vi "TestStand - SetLVFeatureTogglesForBuildAndExecute.vi"(8 "error in":errorcluster, 11 "enable":bool) -> (0 "error out":errorcluster)   [LabVIEW 2023]
panel:
  out "previous value of UseModdateToCheckSourceChanges.Enabled":bool
  out "previous value of AppBuilder.ExportAlwaysIncludedItemsFromPPL":bool
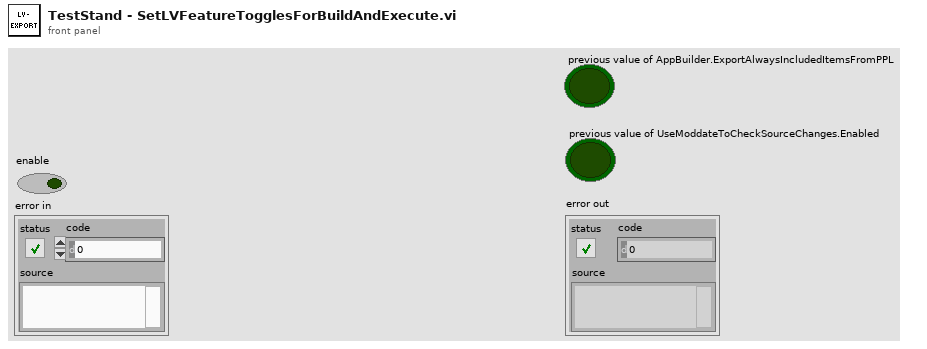
[diagram p1: front panel]
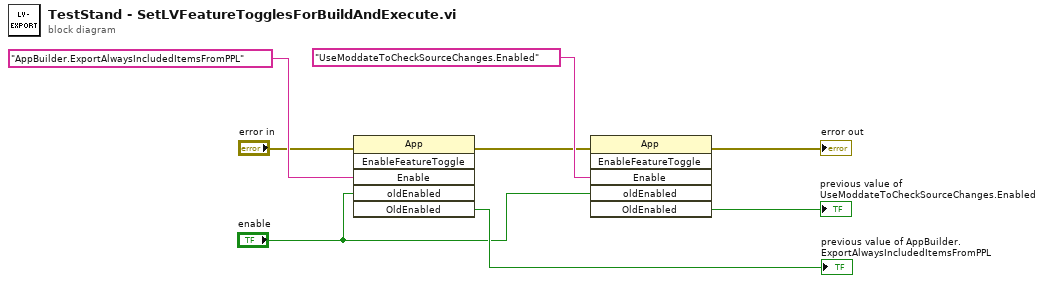
[diagram p0: block diagram]
diagram:
  n1 = invoke class="App" method="EnableFeatureToggle"(error in="error in", "Enable"="AppBuilder.ExportAlwaysIncludedItemsFromPPL" ("TokenName"), "oldEnabled"="enable") -> (error out=w4:errorcluster, "OldEnabled"=→"previous value of AppBuilder.ExportAlwaysIncludedItemsFromPPL":bool)  [unwired: 3 in, 4 out]
  n2 = invoke class="App" method="EnableFeatureToggle"(error in=w4, "Enable"="UseModdateToCheckSourceChanges.Enabled" ("TokenName"), "oldEnabled"="enable") -> (error out=→"error out":errorcluster, "OldEnabled"=→"previous value of UseModdateToCheckSourceChanges.Enabled":bool)  [unwired: 3 in, 4 out]
